vi "Set Platform.vi"(8 "error in (no error)":errorcluster, 10 "Platform":refnum<class "Platform.lvclass">, 11 "PlatformArrayPanel in":refnum<class "PlatformArrayPanel.lvclass">) -> (0 "error out":errorcluster, 3 "PlatformArrayPanel out":refnum<class "PlatformArrayPanel.lvclass">)   [LabVIEW 2020, in "PicoG-App.lvlib" / "PlatformArrayPanel.lvclass"]
uses:
  PlatformArrayPanel.lvclass
  PlatformArrayPanel.lvclass/PlatformArrayPanel.ctl
  Builds/picoG/ppl/PicoG-Core.lvlibp/PicoG-Processor/PicoG-Core/DeployPlatform/Platform.lvclass
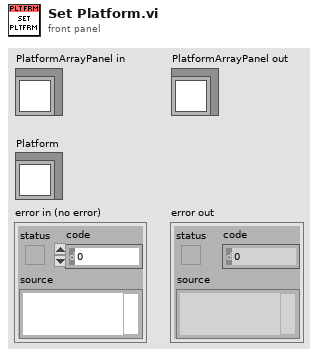
[diagram p1: front panel]
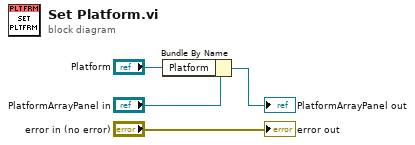
[diagram p0: block diagram]
diagram:
  n1 = Bundle By Name(cluster="PlatformArrayPanel in", "Platform"="Platform") -> (→"PlatformArrayPanel out":refnum<class "PlatformArrayPanel.lvclass">)
  "error out" <- "error in (no error)"
